vi "Create TCP Handler.vi"(8 "error in (no error)":errorcluster, 11 "Volatus Core in":refnum<class "Volatus Core.lvclass">) -> (0 "error out":errorcluster, 3 "Volatus Core out":refnum<class "Volatus Core.lvclass">)   [LabVIEW 2020, in "Volatus.lvlib" / "Volatus Core.lvclass"]
uses:
  Volatus Core.lvclass
  C:/dev/lv20CE/relink/lv-volatus/Volatus/Module/Module.lvclass
  Volatus Core.lvclass/Volatus Core.ctl
  Module/Module.lvclass/Module.ctl
  Remote Messaging Module/Remote Messaging Module.lvclass
  VolatusConfig/VolatusConfigElement/VolatusConfigElement.lvclass
  Vecto Message Bridge/Vecto Message Bridge.lvclass
  C:/dev/lv20CE/relink/lv-vecto/Vecto/TCPMessageHandler/TCPMessageHandler.lvclass
  Module/Module.lvclass
  lv-vecto/Vecto/Vecto/Vecto.lvclass
  lv-vecto/Vecto/TCPMessageService/TCPMessageAPI.lvclass
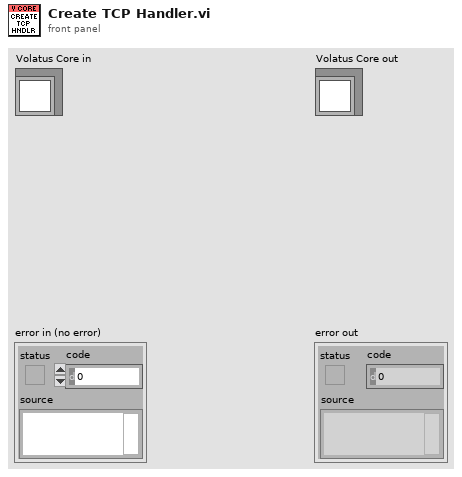
[diagram p1: front panel]
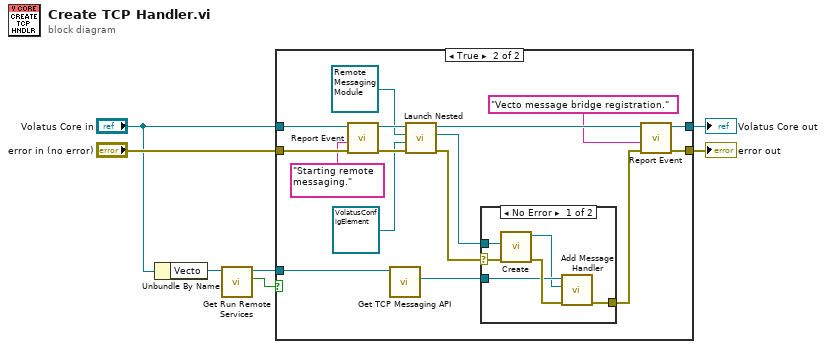
[diagram p0: block diagram]
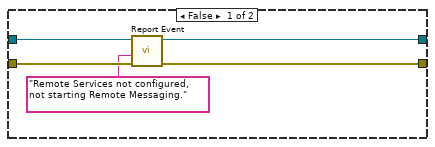
[diagram p2: hidden frame]
diagram:
  n1 = Unbundle By Name("Volatus Core in") -> ("Vecto"=w6:refnum<class "Vecto.lvclass">)
  n2 = call "Get Run Remote Services.vi"("Vecto in"=w6) -> ("Run Remote Services"=w5:bool, "Vecto out"=w4:refnum<class "Vecto.lvclass">)  [unwired: 8 in, 1 out]
  n3 = case shown="True" w5 {
    tunnel: w4 -> [_ w19]
    tunnel: "error in (no error)" -> [w12 w27]
    tunnel: [w11 w15] -> w3
    tunnel: "Volatus Core in" -> [w10 w28]
    tunnel: [w9 w16] -> w1
    frame False {
      n4 = call "Report Event.vi"("error in (no error)"=w12, "Message"="Remote Services not configured, not starting Remote Messaging.", "Module in"=w10) -> ("error out"=w11:errorcluster, "Module out"=w9:refnum<class "Volatus Core.lvclass">)  [unwired: 7 in]
    }
    frame True {
      n5 = call "Report Event.vi"("error in (no error)"=w27, "Message"="Starting remote messaging.", "Module in"=w28) -> ("error out"=w24:errorcluster, "Module out"=w25:refnum<class "Volatus Core.lvclass">)  [unwired: 7 in]
      n6 = call "Get TCP Messaging API.vi"("Vecto in"=w19) -> ("TCP Messaging API"=w18:refnum<class "TCPMessageAPI.lvclass">)  [unwired: 8 in, 2 out]
      n7 = call "Launch Nested.vi"("error in (no error)"=w24, "Config Element"=refnum<class "VolatusConfigElement.lvclass"> refnum, "Nested Module"=refnum<class "Remote Messaging Module.lvclass"> refnum ("Volatus:Remote Messaging Module"), "Parent in"=w25) -> ("error out"=w20:errorcluster, "MessageQ"=w21:refnum<class "MessageQ.lvclass">, "Parent out"=w17:refnum<class "Volatus Core.lvclass">)  [unwired: 5 in]
      n8 = case shown="No Error" w20 {
        selector: w20 -> [w32 w35]
        tunnel: w21 -> [w33 _]
        tunnel: w18 -> [w31 _]
        tunnel: [w29 w35] -> w14
        frame No Error {
          n9 = call "Create.vi"("error in (no error)"=w32, "Remote Messaging"=w33) -> ("error out"=w34:errorcluster, "Vecto Message Bridge out"=w30:refnum<class "Vecto Message Bridge.lvclass">)  [unwired: 8 in]
          n10 = call "Add Message Handler.vi"("error in (no error)"=w34, "TCPMessageHandler"=w30, "TCPMessageAPI in"=w31) -> ("error out"=w29:errorcluster)  [unwired: 7 in, 1 out]
        }
        frame Error {
        }
      }
      n11 = call "Report Event.vi"("error in (no error)"=w14, "Message"="Vecto message bridge registration.", "Module in"=w17) -> ("error out"=w15:errorcluster, "Module out"=w16:refnum<class "Volatus Core.lvclass">)  [unwired: 7 in]
    }
  }
  "error out" <- w3
  "Volatus Core out" <- w1
